vi "testReadArrayFromFileAutoWrapInCluster.vi"(8 "error in (no error)":errorcluster, 11 "TestCase in":refnum<class "EasyXMLTest.lvclass">) -> (0 "error out":errorcluster, 3 "TestCase out":refnum<class "EasyXMLTest.lvclass">)   [LabVIEW 2013, in "EasyXMLTest.lvclass"]
doc: "Verify that error in is not overwritten"
uses:
  EasyXMLTest.lvclass
panel:
  out "LabVIEW Data":variant
  in  "MyArray":string[](array[string])=["foo", "bar"]
  in  "Data to Write":string="<unnamed_cluster>\n  <MyArray>foo</MyArray>\n  <MyArray>bar</MyArray>\n</unnamed_cluster>"
  # "<== Data to Write"
  # "<== XML File"
  # "Parsed Data ==>"
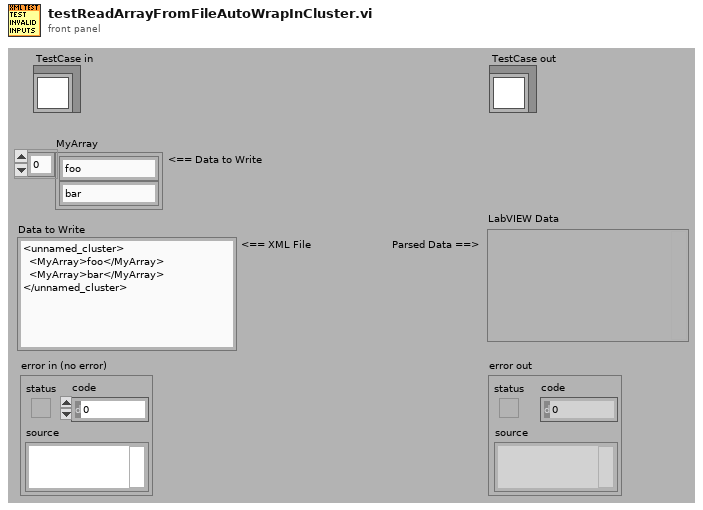
[diagram p1: front panel]
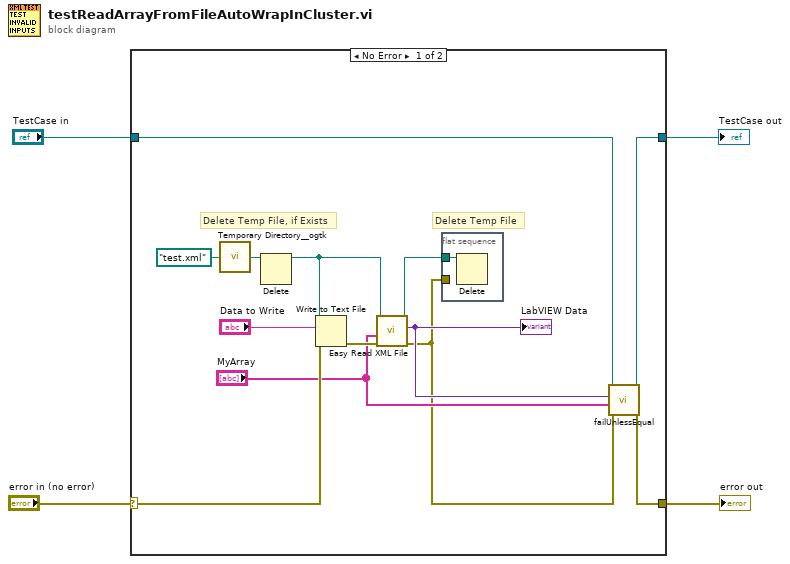
[diagram p0: block diagram]
diagram:
  n1 = case shown="No Error" "error in (no error)" {
    selector: "error in (no error)" -> [w11 w20]
    tunnel: [w13 w20] -> w3
    tunnel: [w14 w19] -> w1
    tunnel: "TestCase in" -> [w15 w19]
    frame No Error {
      # "Delete Temp File"
      # "Delete Temp File, if Exists"
      n2 = call <userlib>:"Temporary Directory__ogtk.vi"("Relative path (.)"=path "test.xml") -> ("Temporary Directory (+ Relative)"=w16:path)
      n3 = Delete(path (use dialog)=w16) -> (deleted path=w9:path)  [unwired: 4 in, 2 out]
      n4 = Write to Text File(file (use dialog)=w9, text="Data to Write", error in=w11) -> (error out=w10:errorcluster)  [unwired: 1 in, 2 out]
      n5 = call "Easy Read XML File.vi"("error in (no error)"=w10, "LabVIEW Data (Type)"="MyArray", "XML File Path"=w9) -> ("error out"=w5:errorcluster, "LabVIEW Data"=w7:variant, "XML File Path (duplicate)"=w8:path)  [unwired: 6 in]
      "LabVIEW Data" <- w7
      n6 = flat-sequence {
        tunnel: w8 -> [w18]
        tunnel: w5 -> [_]
        frame #0 {
          n7 = Delete(path (use dialog)=w18) -> ()  [unwired: 4 in, 3 out]
        }
      }
      n8 = call-dynamic "failUnlessEqual.vi"("error in (no error)"=w5, "y"="MyArray", "x"=w7, "TestCase in"=w15) -> ("error out"=w13:errorcluster, "TestCase out"=w14:refnum<class "EasyXMLTest.lvclass">)  [unwired: 6 in]
    }
    frame Error {
    }
  }
  "error out" <- w3
  "TestCase out" <- w1
